vi "RT Loop - Analyze Acceleration_chopped.vi"(7 "testing":bool, 8 "error in (no error)":errorcluster, 9 "Acceleration RT FIFO In":T1, 10 "FPGA VI Reference Out 2":refnum<k20>, 11 "Message Queue":refnum<queue>) -> (1 "Acceleration RT FIFO Out":T1)   [LabVIEW 2017]
doc: "Read and analyze acceleration waveform data from FPGA via DMA FIFO. If the acceleration is over the limit, then send the acceleration waveform data to the Log Data Loop."
uses:
  UI Error Handlers/support/Message Queue/Message Cluster.ctl
  controls/Acceleration RT FIFO Reference.ctl
  data_sav.ctl
  Control 1.ctl
  Globals/Global - All RT Loop Stop.vi
  Globals/Global - Configuration Options.vi
  <vilib>/Utility/error.llb/Error Cluster From Error Code.vi
  <vilib>/rvi/errors/niLvFpgaAdjustHostInterfaceError.vi
  <vilib>/rvi/interface/nirviMethod/nirviMethod.xnode
  <vilib>/FPGAPlugInAG/Dynamic/niLvFpga_ReadFifo_Dynamic.vi
  <vilib>/rvi/errors/niLvFpgaMergeErrorWithErrorCode.vi
  UI Error Handlers/support/Logging/Logging.lvlib
  UI Error Handlers/support/Message Queue/Message Queue.lvlib
panel:
  out "Free Physical Memory or Largest Contiguous Memory (bytes)":i64(graph)
  out "error out":errorcluster
  out "x-y":u32
  out "G1 status":cluster{"G1 trigger":bool}
  out "G1 status.G1 trigger":bool
  out "sta":bool
  out "logical OR":bool
  in  "Data Rate (Hz)":dbl
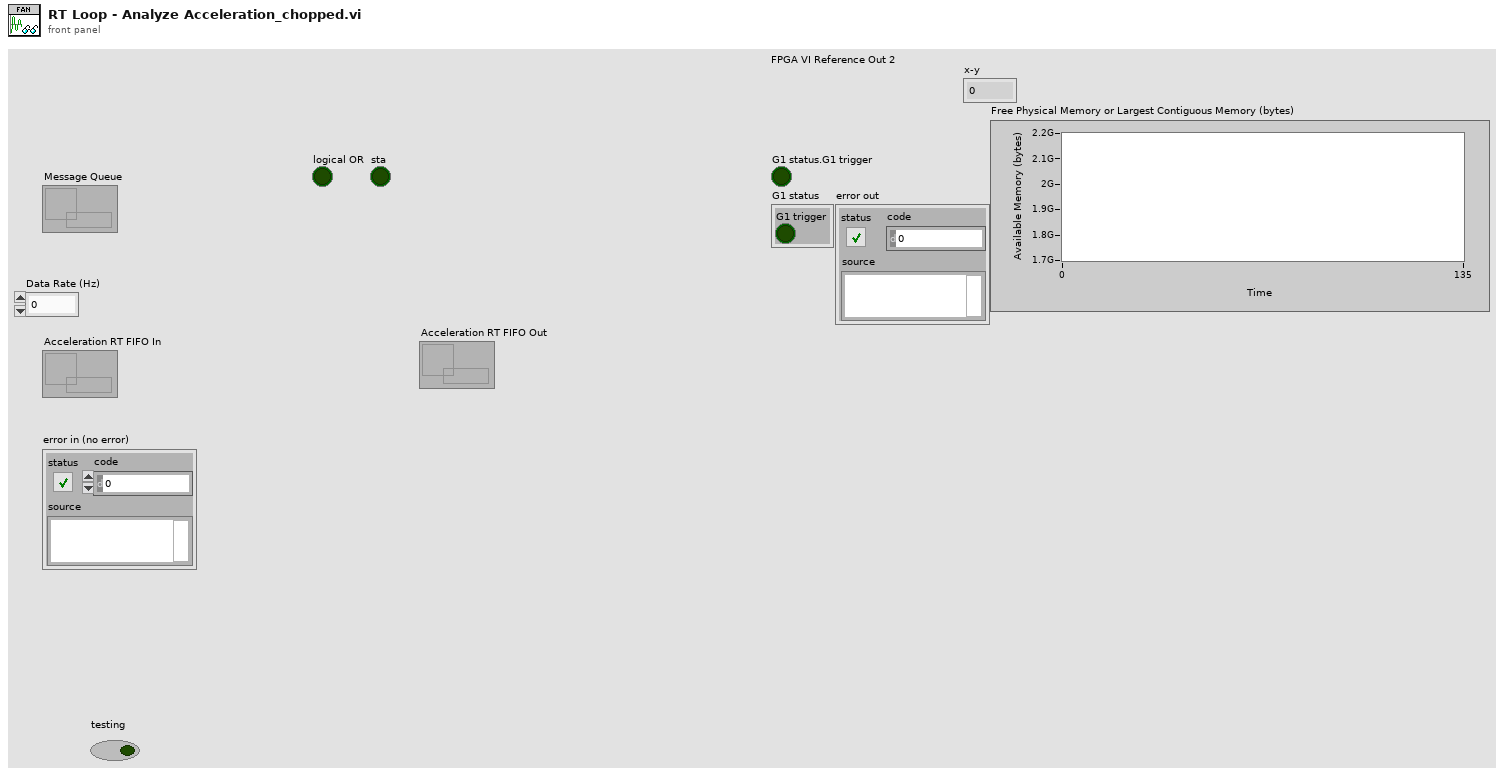
[diagram p1: front panel]
types:
  T1 = typedef "Acceleration RT FIFO Reference.ctl" = refnum<k33>
  T2 = typedef "data_sav.ctl" = cluster{"Log File out 2":refnum<k34>, "Array":T3[]}
  T3 = typedef "Control 1.ctl" = waveform(dbl)
  T4 = cluster{"Tool data":cluster{"Number of teeth":sgl}, "Cutting data":cluster{"rpm":sgl}, "Limits":cluster{"Magnitude threshold":sgl, "Tolerance":sgl}, "G1 status":cluster{"G1 trigger":bool}}
  T5 = cluster{"Log File out":refnum<k34>, waveform(dbl)[]}
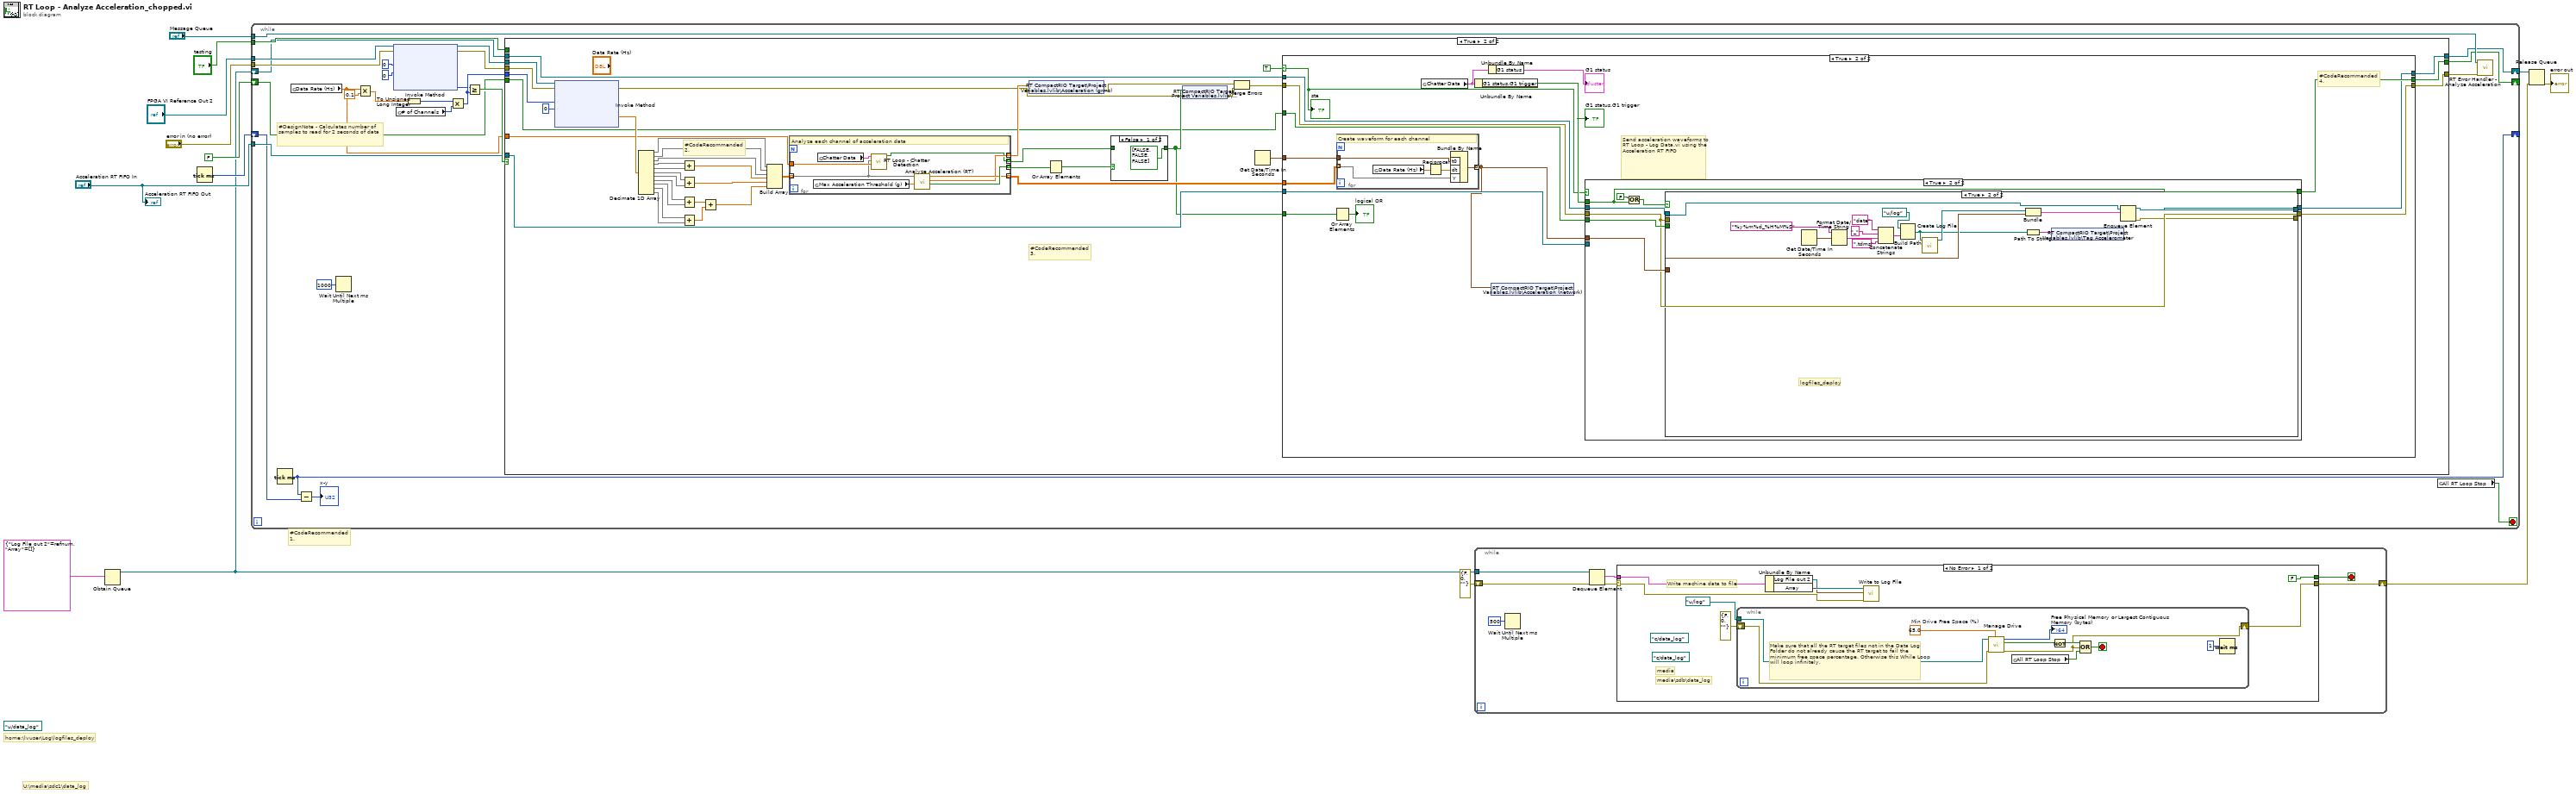
[diagram p0: block diagram]
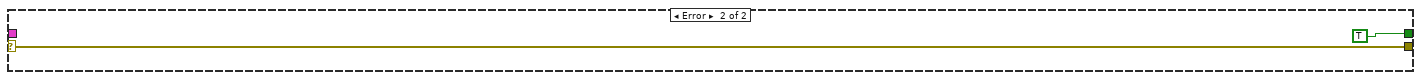
[diagram p2: hidden frame]
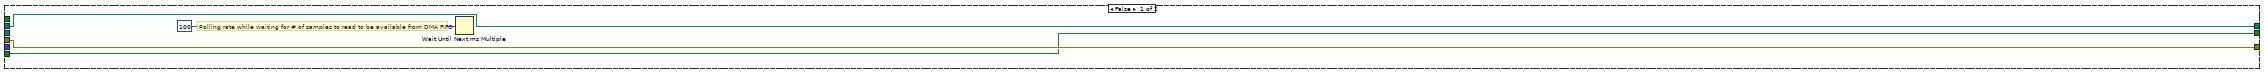
[diagram p3: hidden frame]
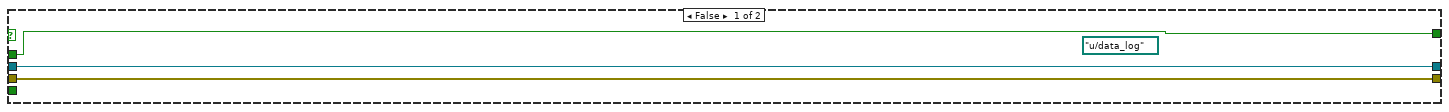
[diagram p6: hidden frame]
diagram:
  (unwired) path "u:/data_log" ("AVI Path")
  # "U:\\media\\sdc1\\data_log"
  # "home:\\lvuser\\Log\\logfiles_deploy"
  # "#CodeRecommended\n1."
  n1 = Obtain Queue(element data type=T2 {"Log File out 2"=refnum, "Array"=[]}) -> (queue out=w5:refnum<queue>)  [unwired: 4 in, 2 out]
  n2 = Tick Count (ms)() -> (millisecond timer value=w8:u32)
  n3 = while {
    tunnel: "FPGA VI Reference Out 2" -> [w40]
    tunnel: "error in (no error)" -> [w39]
    tunnel: "Message Queue" -> [w32]
    tunnel: "Acceleration RT FIFO In" -> [w30]
    tunnel: "testing" -> [w22]
    shift-right: [w21] -> _
    shift-left: FALSE -> [w20]
    shift-right: [w18] -> _
    shift-left: w8 -> [w19]
    shift-right: [w15] -> w4
    shift-left: w5 -> [w16]
    stop <- w33 stop-if-true
    # "#DesignNote - Calculates number of samples to read for 2 seconds of data"
    n4 = Tick Count (ms)() -> (millisecond timer value=w18:u32)
    n5 = global read "Global - Configuration Options.vi" "Data Rate (Hz)"() -> (w24:dbl)
    n6 = Subtract(x=w18, y=w19) -> (x-y=→"x-y":u32)
    n7 = Wait Until Next ms Multiple(millisecond multiple=u32 1000) -> ()  [unwired: 1 out]
    n8 = Multiply(x=w24, y=0.1) -> (x*y=w28:dbl)
    n9 = xnode "Invoke Method"("FPGA VI Reference In"=w40, "error in"=w39, "Number of Elements"=u32 0, "Timeout (ms)"=0) -> ("FPGA VI Reference Out"=w36:refnum<k20>, "error out"=w35:errorcluster, "Elements Remaining"=w23:u32)  [unwired: 1 out]
    n10 = global read "Global - Configuration Options.vi" "# of Channels"() -> (w25:u32)
    n11 = To Unsigned Long Integer(number=w28) -> (unsigned 32bit integer=w27:u32)
    n12 = Multiply(x=w27, y=w25) -> (x*y=w26:u32)
    n13 = Greater Or Equal?(x=w23, y=w26) -> (x >= y?=w34:bool)
    n14 = case shown="True" w34 {
      tunnel: w36 -> [_ w85]
      tunnel: w35 -> [w44 w84]
      tunnel: [w44 w80] -> w31
      tunnel: w26 -> [_ w83]
      tunnel: w30 -> [_ w78]
      tunnel: w24 -> [_ w74]
      tunnel: w22 -> [_ _]
      tunnel: [w42 w66] -> w21
      tunnel: w20 -> [w42 w65]
      tunnel: w16 -> [w41 w49]
      tunnel: [w41 w48] -> w15
      frame False {
        # "Polling rate while waiting for # of samples to read to be available from DMA FIFO"
        n15 = Wait Until Next ms Multiple(millisecond multiple=u32 100) -> ()  [unwired: 1 out]
      }
      frame True {
        # "#CodeRecommended\n3."
        # "#CodeRecommended\n2."
        n16 = xnode "Invoke Method"("FPGA VI Reference In"=w85, "error in"=w84, "Number of Elements"=w83, "Timeout (ms)"=0) -> ("error out"=w73:errorcluster, "Data"=w77:sgl[])  [unwired: 2 out]
        n17 = Decimate 1D Array(w77) -> (w47:sgl[], w62:sgl[], w46:sgl[], w61:sgl[], w60:sgl[], w59:sgl[], w58:sgl[], w57:sgl[], w56:sgl[], w55:sgl[], w54:sgl[])
        n18 = Add(x=w61, y=w60) -> (x+y=w45:sgl[])
        n19 = Add(x=w59, y=w58) -> (x+y=w50:sgl[])
        n20 = Add(x=w57, y=w56) -> (x+y=w53:sgl[])
        n21 = Add(x=w55, y=w54) -> (x+y=w52:sgl[])
        n22 = Add(x=w53, y=w52) -> (x+y=w51:sgl[])
        n23 = Build Array(w47, w62, w46, w45, w50, w51) -> (w63:sgl[][])
        n24 = for {
          tunnel: [w95] -> w79 mode=indexing
          tunnel: [w94] -> w76 mode=indexing
          tunnel: [w93] -> w75 mode=indexing
          tunnel: w74 -> [w91]
          tunnel: [w90] -> w68 mode=indexing
          tunnel: w63 -> [w88] mode=indexing
          # "Analyze each channel of acceleration data"
          n25 = global read "Global - Configuration Options.vi" "Max Acceleration Threshold (g)"() -> (w92:sgl)
          n26 = global read "Global - Configuration Options.vi" "Chatter Data"() -> (w89:T4)
          n27 = call "RT Loop - Chatter Detection.vi"("Data Rate (Hz)"=w91, "Acceleration Waveform (SGL)"=w88, "Chatter Data"=w89) -> ("Chatter?"=w90:bool)  [unwired: 8 in]
          n28 = call "Analyze Acceleration (RT).vi"("Max Instantaneous Acceleration (g)"=w92, "Acceleration Waveform (SGL)"=w88) -> ("Over Limit?"=w95:bool, "Acceleration (grms)"=w93:dbl, "Acceleration Waveform (DBL)"=w94:dbl[])  [unwired: 7 in]
        }
        n29 = shared-variable "RT CompactRIO Target\\Project Variables.lvlib\\Acceleration (grms)"(w75, error in=w73) -> (error out=w71:errorcluster)
        n30 = Or Array Elements(Boolean array=w79) -> (logical OR=w69:bool)
        n31 = case shown="False" w69 {
          tunnel: w68 -> [_ w87]
          tunnel: [bool[] [FALSE, FALSE, FALSE] ("Chatter?") w87] -> w67
          frame False {
          }
          frame True {
          }
        }
        n32 = shared-variable "RT CompactRIO Target\\Project Variables.lvlib\\Chatter?"(w67, error in=w73) -> (error out=w72:errorcluster)
        n33 = Merge Errors(w71, w72) -> (w70:errorcluster)
        n34 = Get Date/Time In Seconds() -> (seconds since 1Jan1904=w81:timestamp)
        n35 = case shown="True" TRUE {
          selector: TRUE -> [_ w100]
          tunnel: w81 -> [_ w114]
          tunnel: w70 -> [w98 w113]
          tunnel: [w98 w103] -> w80
          tunnel: w78 -> [_ w112]
          tunnel: w76 -> [_ w111]
          tunnel: w67 -> [_ w109]
          tunnel: [w97 w106] -> w66
          tunnel: w65 -> [w97 w105]
          tunnel: w49 -> [w96 w102]
          tunnel: [w96 w101] -> w48
          frame False {
          }
          frame True {
            # "#CodeRecommended\n4."
            # "Send acceleration waveforms to RT Loop - Log Data.vi using the Acceleration RT FIFO"
            n36 = Or Array Elements(Boolean array=w109) -> (logical OR=→"logical OR":bool)
            n37 = for {
              tunnel: w111 -> [w148] mode=indexing
              tunnel: w114 -> [w147]
              tunnel: [w145] -> w99 mode=indexing
              # "Create waveform for each channel"
              n38 = global read "Global - Configuration Options.vi" "Data Rate (Hz)"() -> (w144:dbl)
              n39 = Reciprocal(x=w144) -> (1/x=w146:dbl)
              n40 = Bundle By Name("t0"=w147, "dt"=w146, "Y"=w148) -> (w145:waveform(dbl))  [unwired: 1 in]
            }
            n41 = global read "Global - Configuration Options.vi" "Chatter Data"() -> (w108:T4)
            n42 = Unbundle By Name(w108) -> ("G1 status.G1 trigger"=w104:bool)
            "G1 status.G1 trigger" <- w104
            n43 = Unbundle By Name(w108) -> ("G1 status"=→"G1 status":cluster{"G1 trigger":bool})
            n44 = shared-variable "RT CompactRIO Target\\Project Variables.lvlib\\Acceleration (network)"(w99) -> ()  [unwired: 1 in, 1 out]
            n45 = case shown="True" w100 {
              tunnel: w113 -> [w117 w120]
              tunnel: w99 -> [_ w121]
              tunnel: w112 -> [_ _]
              tunnel: w104 -> [w116 w123]
              tunnel: [w116 w123] -> w106
              tunnel: w105 -> [_ w122]
              tunnel: [w117 w120] -> w103
              tunnel: w102 -> [w115 w118]
              tunnel: [w115 w119] -> w101
              frame False {
                (unwired) path "u:/data_log" ("AVI Path")
              }
              frame True {
                n46 = Or(x=FALSE, y=w123) -> (x .or. y?=w125:bool)
                n47 = case shown="True" w125 {
                  tunnel: w122 -> [_ _]
                  tunnel: w121 -> [_ w139]
                  tunnel: w120 -> [w127 _]
                  tunnel: [w127 w142] -> _
                  tunnel: w118 -> [w126 w138]
                  tunnel: [w126 w141] -> w119
                  frame False {
                  }
                  frame True {
                    # "logfiles_deploy"
                    n48 = Get Date/Time In Seconds() -> (seconds since 1Jan1904=w136:timestamp)
                    n49 = Format Date/Time String(time format string (%c)="%y%m%d_%H%M%S", seconds (now)=w136) -> (date/time string=w135:string)  [unwired: 1 out]
                    n50 = Concatenate Strings("data" ("string"), "_" ("string"), w135, ".tdms" ("string")) -> (w137:string)
                    n51 = Build Path(base path=path "u:/log", name or relative path=w137) -> (appended path=w128:path)
                    n52 = call "Create Log File.vi"("Acceleration Exceeded Log Folder"=w128) -> ("Log File out"=w129:refnum<k34>)  [unwired: 9 in, 1 out]
                    n53 = Bundle("Log File out"=w129, w139) -> (w140:T5)  [unwired: 1 in]
                    n54 = Path To String(path=w128) -> (string=w143:string)
                    n55 = shared-variable "RT CompactRIO Target\\Project Variables.lvlib\\Tag Accelerometer"(w143) -> ()  [unwired: 1 in, 1 out]
                    n56 = Enqueue Element(queue=w138, element=w140) -> (queue out=w141:refnum<queue>, error out=w142:errorcluster)  [unwired: 2 in, 1 out]
                  }
                }
              }
            }
            "sta" <- w100
          }
        }
      }
    }
    n57 = global read "Global - All RT Loop Stop.vi" "All RT Loop Stop"() -> (w33:bool)
    n58 = call "RT Error Handler - Analyze Acceleration.vi"("error in (no error)"=w31, "Message Queue"=w32) -> ()  [unwired: 9 in, 1 out]
  }
  n59 = while {
    tunnel: w5 -> [w155]
    shift-right: [w151] -> w3
    shift-left: errorcluster {"status"=FALSE, "code"=0, "source"=""} ("error IO") -> [w154]
    stop <- w152 stop-if-true
    n60 = Wait Until Next ms Multiple(millisecond multiple=u32 500) -> ()  [unwired: 1 out]
    n61 = Dequeue Element(queue=w155, error in (no error)=w154) -> (element=w150:T2, error out=w153:errorcluster)  [unwired: 1 in, 2 out]
    n62 = case shown="No Error" w153 {
      selector: w153 -> [w160 w174]
      tunnel: [FALSE TRUE] -> w152
      tunnel: [w161 w174] -> w151
      tunnel: w150 -> [w159 _]
      frame No Error {
        (unwired) path "c:/data_log" ("AVI Path")
        (unwired) path "c:/data_log" ("AVI Path")
        # "media\\sdb\\data_log"
        # "media"
        # "Write machine data to file"
        n63 = while {
          shift-right: [w168] -> w161
          shift-left: errorcluster {"status"=FALSE, "code"=0, "source"=""} ("error out") -> [w169]
          tunnel: path "u:/log" ("AVI Path") -> [w166]
          stop <- w173 stop-if-true
          w167 = 65.0  # Min Drive Free Space (%)
          # "Make sure that all the RT target files not in the Data Log Folder do not already cause the RT target to fail the minimum free space percentage. Otherwise this While Loop will loop infinitely."
          n64 = call "Manage Drive.vi"("Min Drive Free Space (%)"=w167, "error in"=w169, "Data Folder"=w166) -> ("error out"=w168:errorcluster, "Drive Space Below Limit"=w165:bool, "size (bytes)"=→"Free Physical Memory or Largest Contiguous Memory (bytes)":i64)  [unwired: 6 in]
          n65 = global read "Global - All RT Loop Stop.vi" "All RT Loop Stop"() -> (w170:bool)
          n66 = Not(x=w165) -> (.not. x?=w172:bool)
          n67 = Compound Arithmetic op=OR(w172, w168, w170) -> (w173:bool)
          n68 = Wait (ms)(milliseconds to wait=u32 1) -> ()  [unwired: 1 out]
        }
        n69 = Unbundle By Name(w159) -> ("Log File out 2"=w158:refnum<k34>, "Array"=w157:T3[])
        n70 = call "Write to Log File.vi"("error in (no error)"=w160, "Array of Waveforms"=w157, "Log File in"=w158) -> ()  [unwired: 8 in, 1 out]
      }
      frame Error {
      }
    }
  }
  n71 = Release Queue(queue=w4, error in (no error)=w3) -> (error out=→"error out":errorcluster)  [unwired: 1 in, 2 out]
  "Acceleration RT FIFO Out" <- "Acceleration RT FIFO In"
